vi "Remove Comments(Obsolete).vi"(8 "error in (no error)":errorcluster, 11 "Array":string[](array[string])) -> (0 "error out":errorcluster, 3 "string":string[](array[string]))   [LabVIEW 2019, in "lv-apt-json-file.lvlib"]
uses:
  lv-apt-json-file.lvlib
  <userlib>/_OpenG.lib/array/array.llb/Filter 1D Array (U8)__ogtk.vi
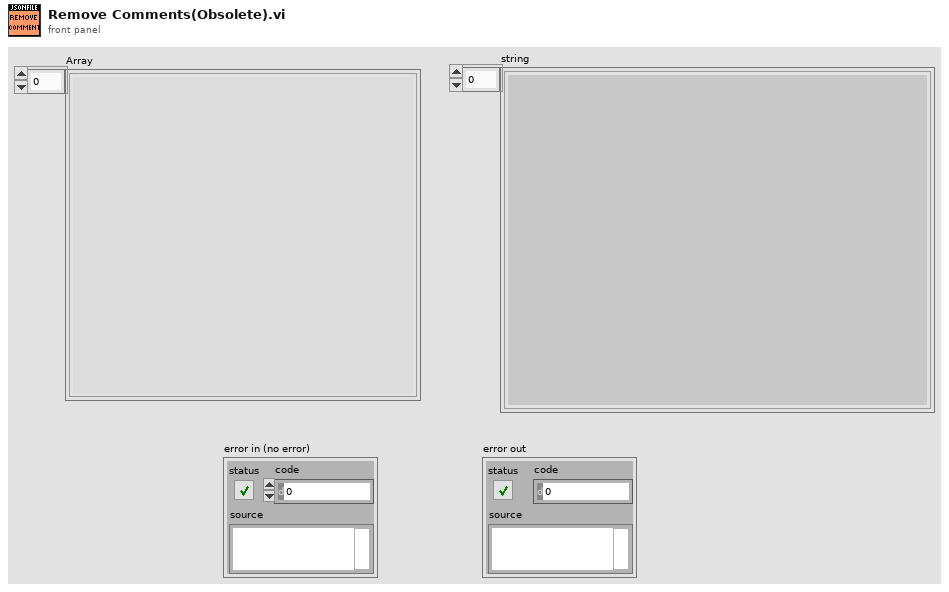
[diagram p1: front panel]
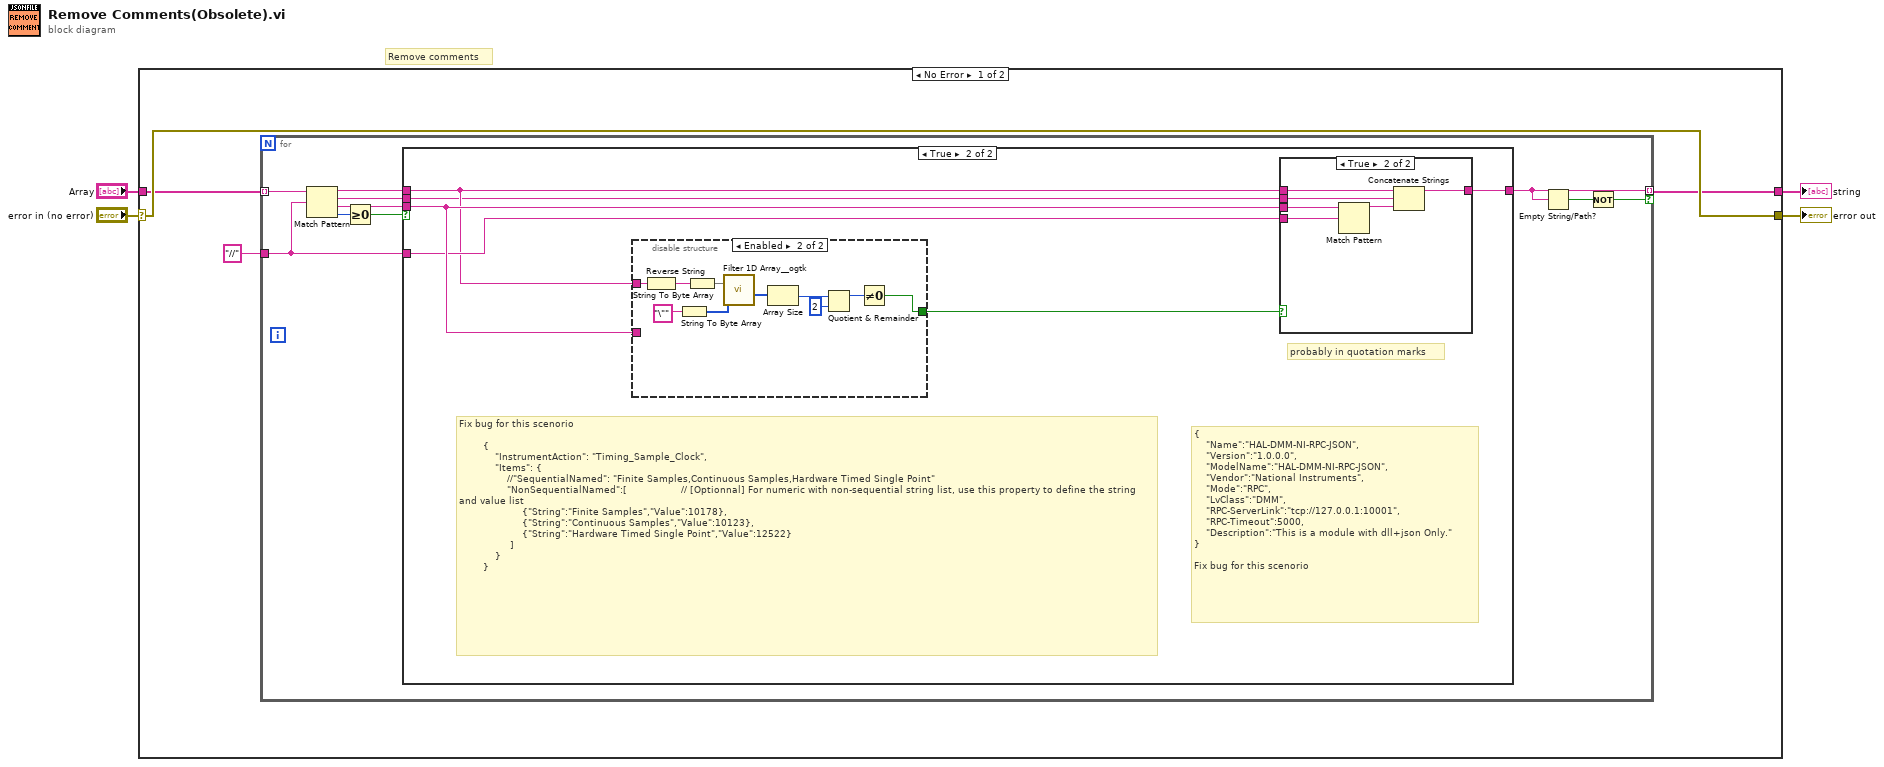
[diagram p0: block diagram]
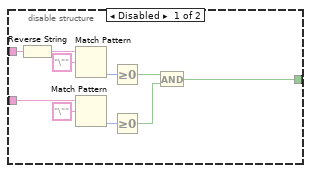
[diagram p3: hidden frame]
diagram:
  # "Remove comments"
  n1 = case shown="No Error" "error in (no error)" {
    selector: "error in (no error)" -> [w7 w53]
    tunnel: "Array" -> [w6 w54]
    tunnel: [w7 w53] -> w2
    tunnel: [w5 w54] -> w1
    frame No Error {
      n2 = for {
        tunnel: w6 -> [w17] mode=indexing
        tunnel: [w12] -> w5 mode=indexing if=w18
        tunnel: "//" ("Annotation Seperator(#)") -> [w9]
        n3 = Match Pattern(string=w17, regular expression=w9) -> (before substring=w13:string, match substring=w10:string, after substring=w11:string, offset past match=w15:i32)  [unwired: 1 in]
        n4 = Greater Or Equal To 0?(x=w15) -> (x >= 0?=w14:bool)
        n5 = case shown="True" w14 {
          tunnel: w13 -> [w19 w23]
          tunnel: [w19 w21] -> w12
          tunnel: w11 -> [_ w25]
          tunnel: w10 -> [_ w22]
          tunnel: w9 -> [_ w24]
          frame False {
          }
          frame True {
            # "Fix bug for this scenorio\n\n        {\n            \"InstrumentAction\": \"Timing_Sample_Clock\",\n            \"Items\": {\n                //\"SequentialNamed\": \"Finite Samples,Continuous Samples,Hardware Timed Single Point\"\n                \"NonSequentialNamed\":[                  // [Optionnal] For numeric with non-sequential string list, use this property to define the string and value list\n                     {\"String\":\"Finite Samples\",\"Value\":10178},\n                     {\"String\":\"Continuous Samples\",\"Value\":10123},\n                     {\"String\":\"Hardware Timed Single Point\",\"Value\":12522}\n                 ]\n            }\n        }"
            # "{\n    \"Name\":\"HAL-DMM-NI-RPC-JSON\",\n    \"Version\":\"1.0.0.0\",\n    \"ModelName\":\"HAL-DMM-NI-RPC-JSON\",\n    \"Vendor\":\"National Instruments\",\n    \"Mode\":\"RPC\",\n    \"LvClass\":\"DMM\",\n    \"RPC-ServerLink\":\"tcp://127.0.0.1:10001\",\n    \"RPC-Timeout\":5000,\n    \"Description\":\"This is a module with dll+json Only.\"\n}\n\nFix bug for this scenorio"
            # "probably in quotation marks"
            n6 = disable-structure shown="Enabled" {
              disable-tunnel: w25 -> [w28 _]
              disable-tunnel: w23 -> [w27 w45]
              disable-tunnel: [w26 w36] -> w20
              frame Disabled {
                n7 = Reverse String(1:w27) -> (0:w35:string)
                n8 = Match Pattern(string=w35, regular expression="\"") -> (offset past match=w32:i32)  [unwired: 1 in, 3 out]
                n9 = Match Pattern(string=w28, regular expression="\"") -> (offset past match=w31:i32)  [unwired: 1 in, 3 out]
                n10 = Greater Or Equal To 0?(x=w32) -> (x >= 0?=w30:bool)
                n11 = Greater Or Equal To 0?(x=w31) -> (x >= 0?=w29:bool)
                n12 = And(x=w30, y=w29) -> (x .and. y?=w26:bool)
              }
              frame Enabled {
                n13 = Reverse String(1:w45) -> (0:w43:string)
                n14 = String To Byte Array(string="\"" ("regular expression")) -> (unsigned byte array=w41:u8[])
                n15 = String To Byte Array(string=w43) -> (unsigned byte array=w44:u8[])
                n16 = call-poly <userlib>:"Filter 1D Array__ogtk.vi"("items to filter"=w41, "array"=w44) -> ("filtered item indices"=w40:i32[])  [unwired: 4 in, 1 out]
                n17 = Array Size(array=w40) -> (size(s)=w39:i32)
                n18 = Quotient & Remainder(x=w39, y=2) -> (x-y*floor(x/y)=w37:i32)  [unwired: 1 out]
                n19 = Not Equal To 0?(x=w37) -> (x != 0?=w36:bool)
              }
            }
            n20 = case shown="True" w20 {
              tunnel: w25 -> [_ w52]
              tunnel: w24 -> [_ w51]
              tunnel: w23 -> [w46 w50]
              tunnel: w22 -> [_ w49]
              tunnel: [w46 w47] -> w21
              frame False {
              }
              frame True {
                n21 = Match Pattern(string=w52, regular expression=w51) -> (before substring=w48:string)  [unwired: 1 in, 3 out]
                n22 = Concatenate Strings(w50, w49, w48) -> (w47:string)
              }
            }
          }
        }
        n23 = Empty String/Path?(string/path=w12) -> (empty?=w16:bool)
        n24 = Not(x=w16) -> (.not. x?=w18:bool)
      }
    }
    frame Error {
    }
  }
  "string" <- w1
  "error out" <- w2
